vi "PH_DIM.add String Array Service.vi"(0 "i ref in":refnum<vi>, 1 "Service Name":string="N/A", 2 "String Array":string[](array[string]), 5 "error in (no error)":errorcluster) -> (14 "i ref out":refnum<vi>, 17 "Service ID":i32, 19 "error out":errorcluster)   [LabVIEW 2014, in "PH_Common.lvlib"]
doc: "This VI publishes an array of strings opening a service \"<instancename>_ServiceName\", if no error comes in, the array size is not 0 and the Service Name is not N/A. For further use, the Service ID is given out (it is \"-1\" if the service has not been added)."
uses:
  PH_Common.lvlib
  lib.lib/DimLVEvent/LVDimInterface/LVDimInterface.lvlib
  CSCore/CSSystem/CSSystemLib/CSSystemLib.lvlib
  CSCore/CSSystem/CoreLib/CoreLib.lvlib
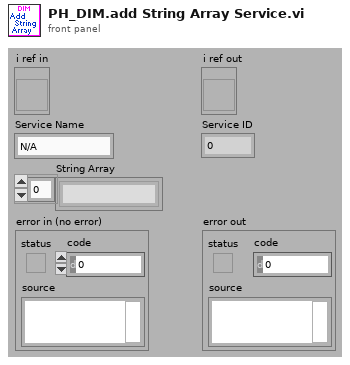
[diagram p1: front panel]
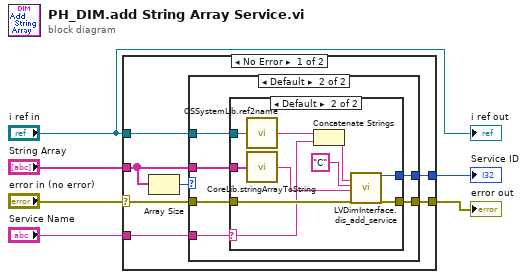
[diagram p0: block diagram]
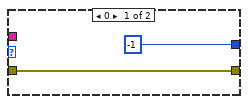
[diagram p2: hidden frame]
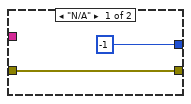
[diagram p3: hidden frame]
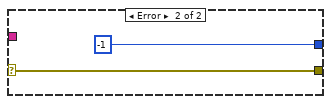
[diagram p4: hidden frame]
diagram:
  n1 = case shown="No Error" "error in (no error)" {
    selector: "error in (no error)" -> [w10 w35]
    tunnel: [w13 -1 ("my_serviceID")] -> w6
    tunnel: [w12 w35] -> w5
    tunnel: "String Array" -> [w9 _]
    tunnel: "i ref in" -> [w11 _]
    tunnel: "Service Name" -> [w7 _]
    frame No Error {
      n2 = Array Size(array=w9) -> (size(s)=w8:i32)
      n3 = case shown="Default" w8 {
        tunnel: [-1 ("my_serviceID") w21] -> w13
        tunnel: [w15 w20] -> w12
        tunnel: w11 -> [_ w19]
        tunnel: w10 -> [w15 w18]
        tunnel: w9 -> [_ w17]
        tunnel: w7 -> [_ w16]
        frame 0 {
        }
        frame Default {
          n4 = case shown="Default" w16 {
            selector: w16 -> [_ w24]
            tunnel: [-1 ("my_serviceID") w33] -> w21
            tunnel: [w23 w32] -> w20
            tunnel: w19 -> [_ w27]
            tunnel: w18 -> [w23 w26]
            tunnel: w17 -> [_ w25]
            frame "N/A" {
            }
            frame Default {
              n5 = call "CSSystemLib.ref2name.vi"("obj refnum"=w27) -> ("name"=w28:string)
              n6 = call "CoreLib.stringArrayToString.vi"("Array"=w25) -> ("String"=w31:string)
              n7 = Concatenate Strings(w28, w24) -> (w29:string)
              n8 = call "LVDimInterface.dis_add_service.vi"("serviceName"=w29, "typeDescriptor"="C", "data"=w31, "error in (no error)"=w26) -> ("my_serviceID"=w33:i32, "error out"=w32:errorcluster)  [unwired: 14 in]
            }
          }
        }
      }
    }
    frame Error {
    }
  }
  "Service ID" <- w6
  "error out" <- w5
  "i ref out" <- "i ref in"
